vi "Test - Obtain Known Object Target.vi"() -> ()   [LabVIEW 2019]
doc: "This VI serves as the target VI for the Obtaining Known Object Reference.vi example, which opens a reference to the Edit me control and changes the Representation of the control to I32.\n\nDo not save changes to this VI."
panel:
  out "Array output":ext[](array[numeric])
  in  "Control":dbl
  in  "Edit me":dbl
  in  "Iterations":i32
  # "Select Help>>Show Context Help and move the cursor over the VI icon to display help for this VI.\n\nDO NOT SAVE CHANGES TO THIS VI. This VI serves as the target for the Obtaining Known Object Reference.vi example. Therefore, changing this VI might prevent the Obtaining Known Object Reference.vi example from demonstrating its scripting task."
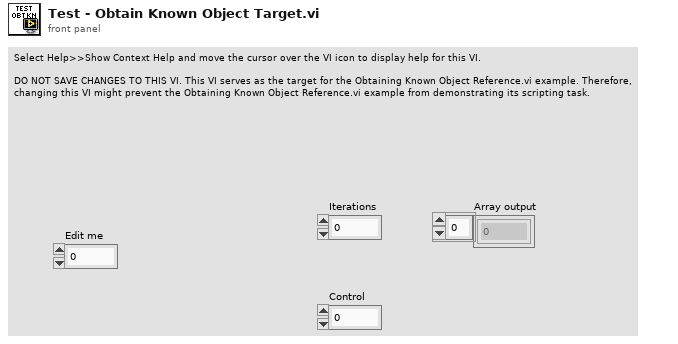
[diagram p1: front panel]
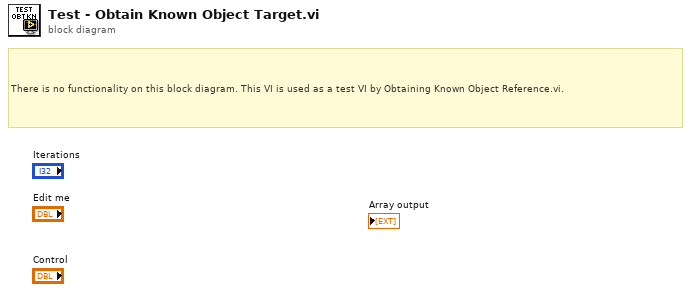
[diagram p0: block diagram]
diagram:
  # "There is no functionality on this block diagram. This VI is used as a test VI by Obtaining Known Object Reference.vi."
